vi "Read File Chunk to copy.vi"(8 "error in":errorcluster, 9 "Length to copy":i32, 10 "Start index":i64, 11 "refnum":refnum<file>) -> (0 "error out":errorcluster, 1 "File body to copy":string, 3 "refnum out":refnum<file>)   [LabVIEW 2018]
panel:
  out "offset (in bytes)":i64
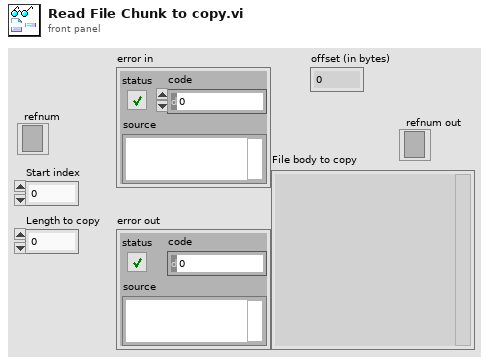
[diagram p1: front panel]
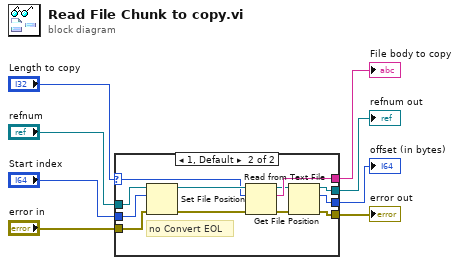
[diagram p0: block diagram]
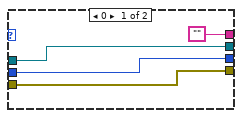
[diagram p2: hidden frame]
diagram:
  n1 = case shown="1, Default" "Length to copy" {
    selector: "Length to copy" -> [_ w13]
    tunnel: "Start index" -> [w11 w22]
    tunnel: "refnum" -> [w10 w21]
    tunnel: ["" w20] -> w6
    tunnel: "error in" -> [w9 w19]
    tunnel: [w10 w17] -> w4
    tunnel: [w9 w15] -> w3
    tunnel: [w11 w14] -> w2
    frame 0 {
    }
    frame 1, Default {
      # "no Convert EOL"
      n2 = Set File Position(offset (in bytes) (0)=w22, refnum=w21, error in=w19) -> (refnum out=w23:refnum<file>, error out=w24:errorcluster)  [unwired: 1 in]
      n3 = Read from Text File(file (use dialog)=w23, count=w13, error in=w24) -> (refnum out=w18:refnum<file>, text=w20:string, error out=w16:errorcluster)  [unwired: 1 in, 1 out]
      n4 = Get File Position(4:w16, 7:w18) -> (0:w15:errorcluster, 2:w14:i64, 3:w17:refnum<file>)
    }
  }
  "File body to copy" <- w6
  "refnum out" <- w4
  "error out" <- w3
  "offset (in bytes)" <- w2
